vi "Acquire Image.vi"(8 "error in (no error)":errorcluster, 9 "Cluster":T1={"Bayer"={"Algorithm"=0, "Gain R"=1.0, "Gain B"=1.0, "Gain G"=1.0, "Pattern"=5}, "Acquisition Control"={"Trigger Selector"=0, "Acquisition Frame Rate"=0.0, "Exposure Time"=0.0, "Acquisition Frame Rate Target"=0.0}, "Analog Control"={"Black Level"=1.5, "Gain Selector"=10, "Gain"=1.0}} {"Analog Control"."Gain" min=1.0 max=15.0; "Analog Control"."Gain Selector" items=["Analog All"=10, "Digital All"=20]; "Analog Control"."Black Level" min=0.0 max=255.9375; "Acquisition Control"."Acquisition Frame Rate Target" min=0.001 max=150000000.0; "Acquisition Control"."Exposure Time" min=27.793333333333333 max=1048539.7933333333; "Acquisition Control"."Acquisition Frame Rate" min=0.9536888685435264 max=30.757874015748033; "Acquisition Control"."Trigger Selector" items=["Frame Start"=3, "Exposure Start"=10]; "Bayer"."Pattern" items=["Use hardware value"=5, "None"=0, "GB"=1, "GR"=2, "BG"=3, "RG"=4]; "Bayer"."Gain G" min=0.0 max=3.999; "Bayer"."Gain B" min=0.0 max=3.999; "Bayer"."Gain R" min=0.0 max=3.999; "Bayer"."Algorithm" items=["Bilinear", "VNG"]}, 10 "Stop":bool, 11 "Camera in":refnum<class "Camera.lvclass">) -> (0 "error out":errorcluster, 2 "Image Out":T2(plugin-control), 3 "Camera out":refnum<class "Camera.lvclass">)   [LabVIEW 2021, in "Camera.lvclass"]
uses:
  Camera.lvclass
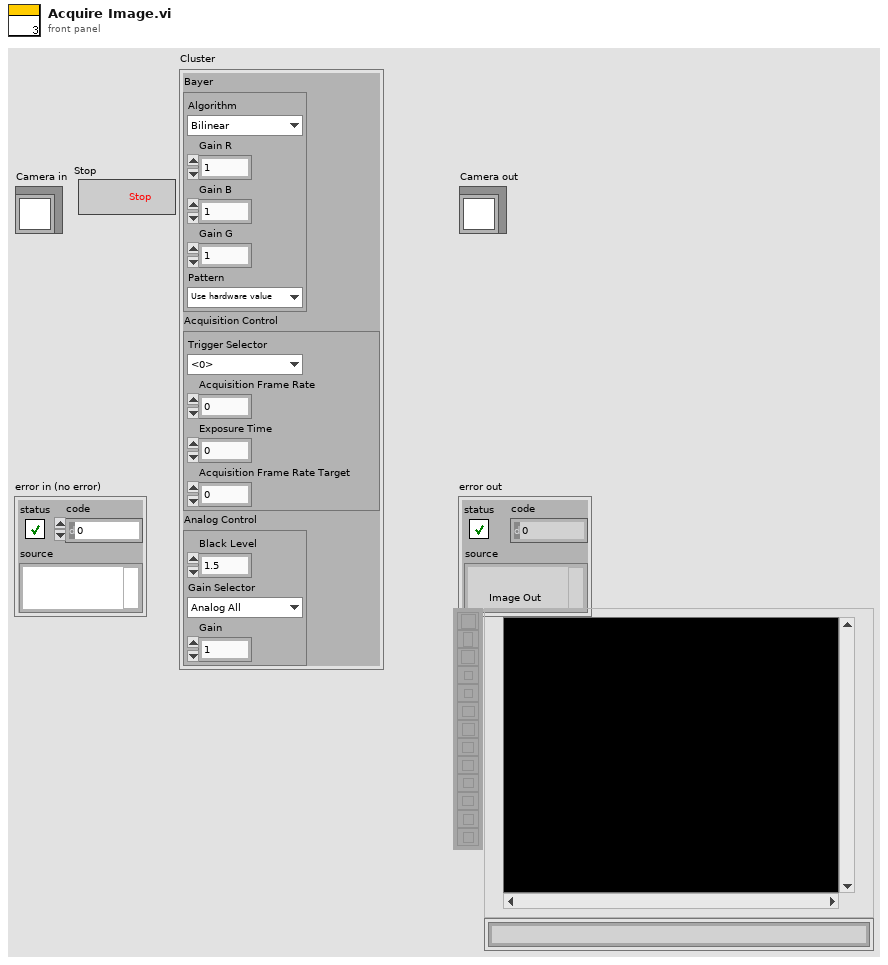
[diagram p1: front panel]
types:
  T1 = cluster{"Bayer":cluster{"Algorithm":u32, "Gain R":dbl, "Gain B":dbl, "Gain G":dbl, "Pattern":u32}, "Acquisition Control":cluster{"Trigger Selector":u32, "Acquisition Frame Rate":dbl, "Exposure Time":dbl, "Acquisition Frame Rate Target":dbl}, "Analog Control":cluster{"Black Level":dbl, "Gain Selector":u32, "Gain":dbl}}
  T2 = typedef "IMAQ Image.ctl" = refnum<image>
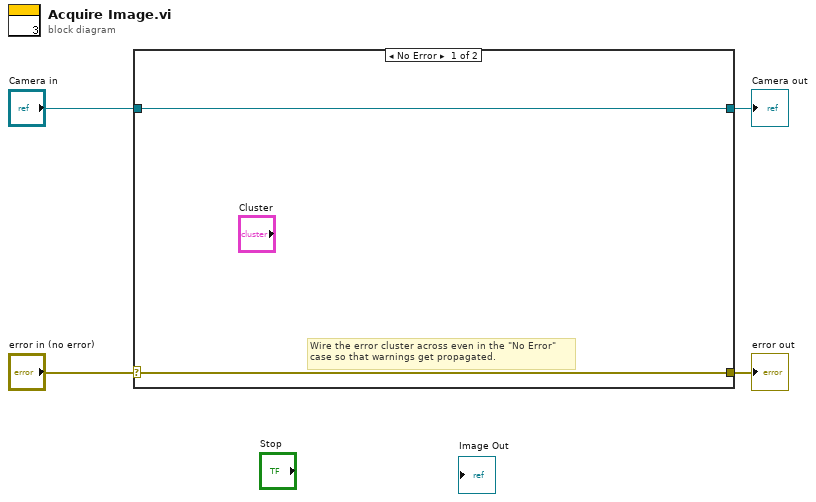
[diagram p0: block diagram]
diagram:
  n1 = case shown="No Error" "error in (no error)" {
    selector: "error in (no error)" -> [w5 w8]
    tunnel: [w5 w8] -> w3
    tunnel: [w6 w7] -> w1
    tunnel: "Camera in" -> [w6 w7]
    frame No Error {
      # "Wire the error cluster across even in the \"No Error\"\ncase so that warnings get propagated."
    }
    frame Error {
    }
  }
  "error out" <- w3
  "Camera out" <- w1
